vi "Check Error.vi"(8 "error in (no error)":errorcluster, 11 "queue in":refnum<queue>) -> (0 "error out":errorcluster, 3 "queue out":refnum<queue>)   [LabVIEW 2017, in "Shared Variables CD 2.0 Configuration.lvlib"]
uses:
  Shared Variables CD 2.0 Configuration.lvlib
  Channel Configuration States.ctl
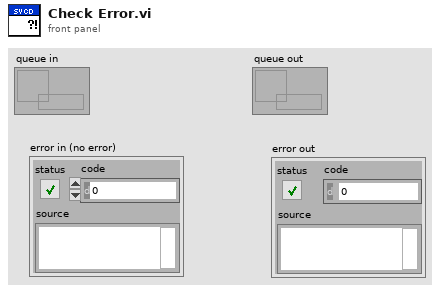
[diagram p1: front panel]
types:
  T1 = typedef "Shared Variables CD 2.0 Configuration.lvlib/Channel Configuration States.ctl" = enum16{"Open/Init", "Start Update", "Get VS Channels", "Get Available Ch from Target", "Wait On User Action", "Update Target Tree", "Update VS Trees", "Update Done", "Create VS Channels", "Remove VS Channels", "Error", "Close"}
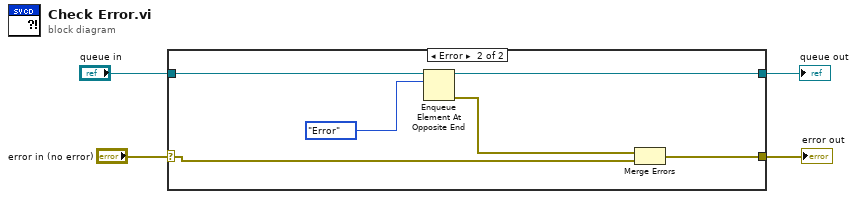
[diagram p0: block diagram]
diagram:
  n1 = case shown="Error" "error in (no error)" {
    selector: "error in (no error)" -> [w6 w10]
    tunnel: [w6 w12] -> w3
    tunnel: "queue in" -> [w5 w11]
    tunnel: [w5 w8] -> w1
    frame No Error {
    }
    frame Error {
      n2 = Enqueue Element At Opposite End(queue=w11, element=Channel_Configuration_States."Error") -> (queue out=w8:refnum<queue>, error out=w7:errorcluster)  [unwired: 2 in, 1 out]
      n3 = Merge Errors(w7, w10) -> (w12:errorcluster)
    }
  }
  "error out" <- w3
  "queue out" <- w1
